vi "Do.vi"(6 "Input":variant, 8 "error in":errorcluster, 9 "Self Enqueuer":refnum<class "Message Enqueuer.lvclass">, 10 "Series Enqueuer":refnum<class "Message Enqueuer.lvclass">, 11 "Sample Airtemp PWM Control in":refnum<class "Sample Airtemp PWM Control.lvclass">) -> (0 "error out":errorcluster, 3 "Sample Airtemp PWM Control out":refnum<class "Sample Airtemp PWM Control.lvclass">)   [LabVIEW 2023, in "Sample Airtemp PWM Control.lvclass"]
uses:
  Sample Airtemp PWM Control.lvclass
  <vilib>/ActorFramework/Message Enqueuer/Message Enqueuer.lvclass
  Task/Task Base/Task Base.lvclass/Task Base.ctl
  Sample Airtemp PWM Control.lvclass/Sample Airtemp PWM Control.ctl
  Task/Task Base/Task Base.lvclass
  Measure and Stimulus Subsystems/Measure and Stimulus Subsystems.lvclass
  D:/git/HAL/HAL GOOP4/Task/Task Base/Task Base.lvclass
  D:/git/HAL/HAL GOOP4/Tests/RT Tests/Sample Tasks/Sample Airtemp PWM Control/Sample Airtemp PWM Control.lvclass
panel:
  out "Process Variable":dbl
  out "Control Output":dbl format="%.2f"
  out "Setpoint":dbl
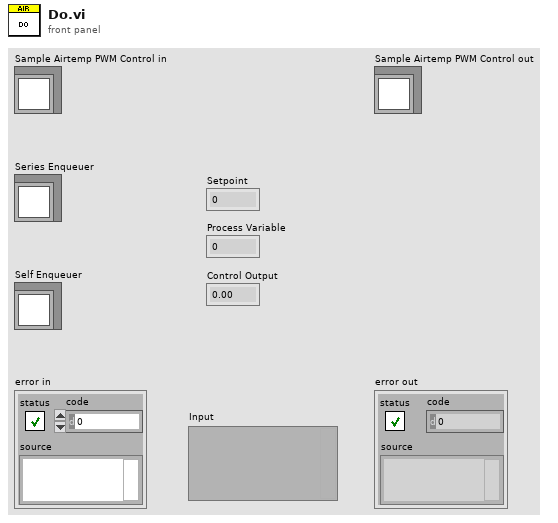
[diagram p1: front panel]
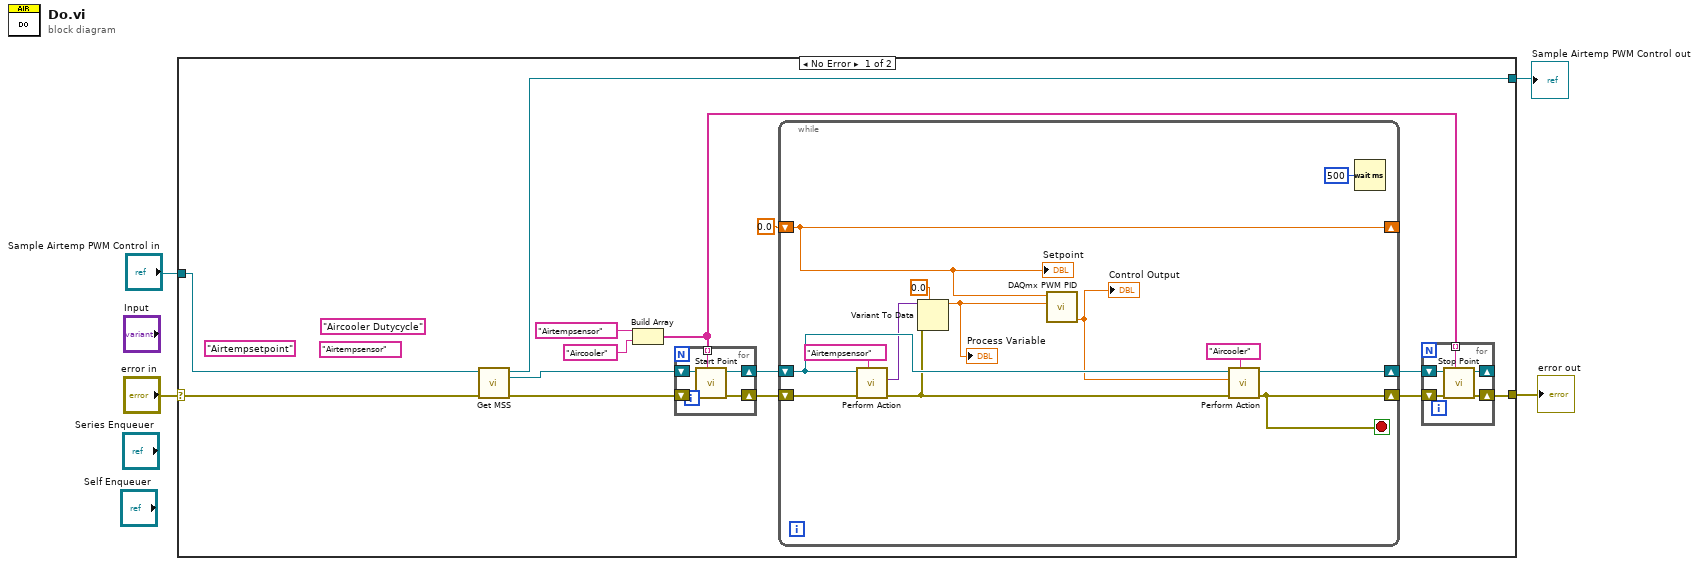
[diagram p0: block diagram]
diagram:
  n1 = case shown="No Error" "error in" {
    selector: "error in" -> [w15 w43]
    tunnel: [w11 w43] -> w1
    tunnel: [w7 w42] -> w2
    tunnel: "Sample Airtemp PWM Control in" -> [w6 w42]
    frame No Error {
      (unwired) "Aircooler Dutycycle" ("Target Name")
      (unwired) "Airtempsetpoint" ("Target Name")
      (unwired) "Airtempsensor" ("Target Identifier")
      n2 = call "Get MSS.vi"("error in (no error)"=w15, "Task Base in"=w6) -> ("error out"=w14:errorcluster, "MSS"=w13:refnum<class "Measure and Stimulus Subsystems.lvclass">, "Task Base out"=w7:refnum<class "Sample Airtemp PWM Control.lvclass">)  [unwired: 7 in]
      n3 = Build Array("Airtempsensor" ("Target Identifier"), "Aircooler" ("Target Identifier")) -> (w8:string[])
      n4 = for {
        shift-right: [w23] -> w18
        shift-left: w14 -> [w21]
        shift-right: [w22] -> w17
        shift-left: w13 -> [w20]
        tunnel: w8 -> [w19] mode=indexing
        n5 = call "Start Point.vi"("Point Ident"=w19, "error in"=w21, "MSS in"=w20) -> ("error out"=w23:errorcluster, "MSS out"=w22:refnum<class "Measure and Stimulus Subsystems.lvclass">)  [unwired: 7 in]
      }
      n6 = while {
        shift-right: [w26] -> w16
        shift-left: w18 -> [w32]
        shift-right: [w34] -> w12
        shift-left: w17 -> [w31]
        shift-right: [w27] -> _
        shift-left: 0.0 -> [w27]
        stop <- w26 stop-if-true
        n7 = call "Perform Action.vi"("Point Ident"="Airtempsensor" ("Target Identifier"), "error in"=w32, "MSS in"=w31) -> ("error out"=w28:errorcluster, "Output"=w29:variant)  [unwired: 6 in, 1 out]
        n8 = Variant To Data(error in=w28, type=0.0, Variant=w29) -> (data=w25:dbl)  [unwired: 1 out]
        "Process Variable" <- w25
        n9 = call "DAQmx PWM PID.vi"("Process Variable"=w25, "Setpoint"=w27) -> ("Control Output"=w24:dbl)  [unwired: 9 in]
        "Control Output" <- w24
        n10 = call "Perform Action.vi"("Point Ident"="Aircooler" ("Target Ident"), "error in"=w28, "Input"=w24, "MSS in"=w31) -> ("error out"=w26:errorcluster, "MSS out"=w34:refnum<class "Measure and Stimulus Subsystems.lvclass">)  [unwired: 5 in, 1 out]
        n11 = Wait (ms)(milliseconds to wait=u32 500) -> ()  [unwired: 1 out]
        "Setpoint" <- w27
      }
      n12 = for {
        shift-right: [w39] -> w11
        shift-left: w16 -> [w41]
        tunnel: w8 -> [w37] mode=indexing
        shift-right: [w38] -> _
        shift-left: w12 -> [w40]
        n13 = call "Stop Point.vi"("Point Ident"=w37, "error in"=w41, "MSS in"=w40) -> ("error out"=w39:errorcluster, "MSS out"=w38:refnum<class "Measure and Stimulus Subsystems.lvclass">)  [unwired: 7 in]
      }
    }
    frame Error {
    }
  }
  "error out" <- w1
  "Sample Airtemp PWM Control out" <- w2
